vi "Periodic Tasks.vi"(8 "error in":errorcluster) -> ()   [LabVIEW 2018]
doc: "This VI runs in parallel to other tasks. It can contain as many user-defined periodic loops as you need. These can carry out PID or other sorts of timed response."
uses:
  PWF_Venom_LabVIEW/Public/TypeDefs/PwF_Venom_PIDParams.ctl
  DriveVenomDevRefs.ctl
  <vilib>/Rock Robotics/WPI/MotorControl/WPI_MotorControlDeviceRef.ctl
  <vilib>/Rock Robotics/WPI/MotorControl/WPI_MotorControlType.ctl
  <vilib>/Rock Robotics/SystemInterfaces/DIO/FPGA_DIOPWMChannel.ctl
  <vilib>/Rock Robotics/WPI/PWM/WPI_PWMDeadband.ctl
  <vilib>/Rock Robotics/SystemInterfaces/DIO/FPGA_DIOChannel.ctl
  DriveState.ctl
  PWF_Venom_LabVIEW/Public/TypeDefs/PwF_Venom_ControlMode.ctl
  88a8256b-dd6c-4d38-b021-9946be483166.vi
  72a4271e-8a2f-4e63-bef0-ab0047b3c302.vi
  4419bb08-cace-4eec-81e3-431b0f19f77f.vi
  43bb15c8-37b4-49b3-9761-3a694f89d06e.vi
  681b6e5e-4677-4682-a16d-7f94549bf0f7.vi
  f8245736-c666-4745-b76e-80ca56998d75.vi
  eff852b5-78a3-4797-aee6-6215f14f6dac.vi
  <vilib>/Array/Sort 2D Array - Pop Stack.vi
  <vilib>/Array/Sort 2D Array - Push Stack.vi
  <vilib>/Rock Robotics/WPI/Utilities/WPI_GetSetVariantRefNum.vi
  <vilib>/Rock Robotics/WPI/ThirdParty/Phoenix-LabVIEW/Pigeon IMU/CTRE_PigeonIMU_GetFusedHeading.vi
  <vilib>/Rock Robotics/Network Tables/NT Read Numeric Array.vi
  PWF_Venom_LabVIEW/PwF_Venom.lvlib
panel:
  in  "Set Angle":dbl(slide) scale=-180.0..180.0
  out "Degrees Off":dbl
  out "Center":dbl
  out "Height":dbl
  in  "Offset":dbl=182.0
  out "Waveform Chart":dbl(graph)=-0.0
  in  "PID Params":T1={"kP"=0.5, "kI"=0.0, "kD"=0.0, "kF"=0.184, "b"=0.0}
  in  "Track Width":dbl=2.3125
  in  "Tuning":dbl=10.0
  in  "Min Turn Radius":dbl=1.0
  in  "Max Wheel Velocity":dbl=4.0
  out "Avg Left Encoder (ft/s)":dbl
  out "Left Encoder (ft/s)":dbl
  in  "MinPower":dbl=0.063 format="%#_13g"
  out "dTime":u32=31
  out "Speed":dbl
  out "Position":dbl=-0.008333333333333333
  out "XY Graph":cluster{dbl[], dbl[]}(graph)
  out "RightEncoderInches":dbl=0.005423177083333334
  out "LeftEncoderInches":dbl=0.037962239583333335
  out "RightEncoderRaw":dbl=0.25
  out "LeftEncoderRaw":dbl=1.75
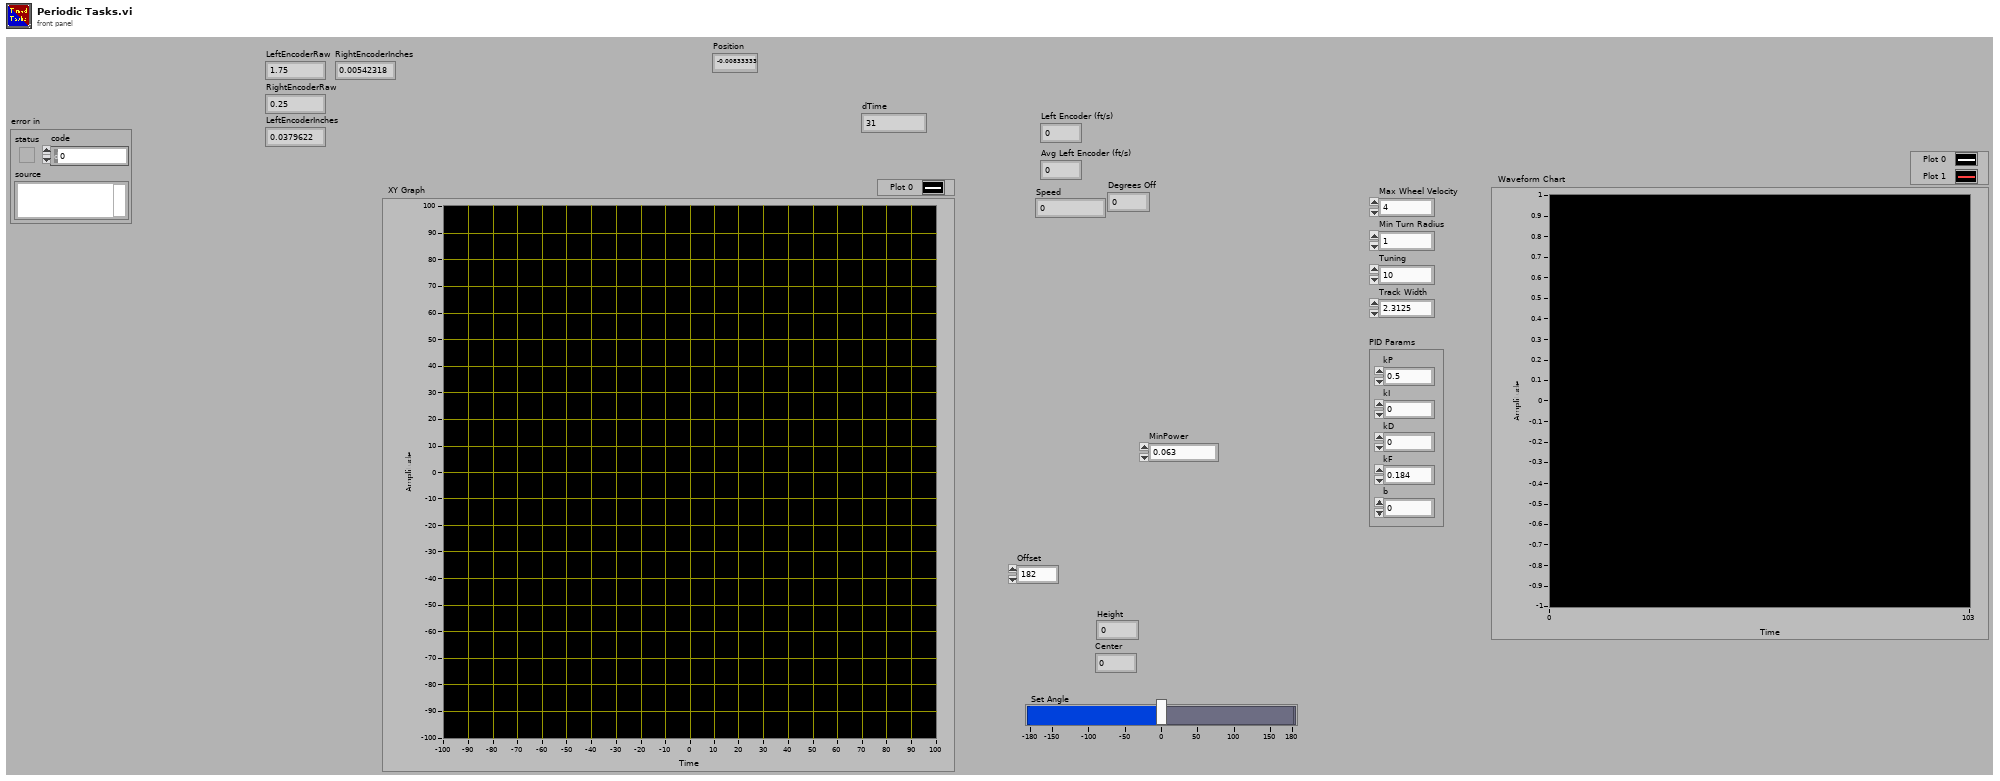
[diagram p1: front panel]
types:
  T1 = typedef "PwF_Venom.lvlib/PwF_Venom_PIDParams.ctl" = cluster{"kP":dbl, "kI":dbl, "kD":dbl, "kF":dbl, "b":dbl}
  T2 = cluster{"millisecond timer value":u32, "Distance":dbl}
  T3 = typedef "DriveVenomDevRefs.ctl" = cluster{"FrontLeft":T4, "FrontRight":T4}
  T4 = typedef "WPI_MotorControlDeviceRef.ctl" = cluster{"DeviceStatus":errorcluster, "Type":T5, "PWM":cluster{"PWM Channel":T6, "DeadBand":T7}, "CAN":cluster{"Device Number":u8, "SetOutput VI Ref":variant, "GetOutput VI Ref":variant, "Enable VI Ref":variant, "Disable VI Ref":variant, "Data":variant}, "Invert":bool, "DIO PWM":cluster{"PWM \"Enable\" Channel":T6, "DIOChannel":T8, "PWM Rate":dbl}}
  T5 = typedef "WPI_MotorControlType.ctl" = enum16{"PWM", "CAN", "DIO PWM"}
  T6 = typedef "FPGA_DIOPWMChannel.ctl" = enum8{"PWM 0", "PWM 1", "PWM 2", "PWM 3", "PWM 4", "PWM 5", "PWM 6", "PWM 7", "PWM 8", "PWM 9", "PWM MXP 0", "PWM MXP 1", "PWM MXP 2", "PWM MXP 3", "PWM MXP 4", "PWM MXP 5", "PWM MXP 6", "PWM MXP 7", "PWM MXP 8", "PWM MXP 9", "Invalid"}
  T7 = typedef "WPI_PWMDeadband.ctl" = cluster{"Name":string, "maxPositivePwm":i32, "minPositivePwm":i32, "centerPwm":i32, "maxNegativePwm":i32, "minNegativePwm":i32, "angularRange":u16}
  T8 = typedef "FPGA_DIOChannel.ctl" = enum8{"DIO 0", "DIO 1", "DIO 2", "DIO 3", "DIO 4", "DIO 5", "DIO 6", "DIO 7", "DIO 8", "DIO 9", "DIO MXP 0", "DIO MXP 1", "DIO MXP 2", "DIO MXP 3", "DIO MXP 4", "DIO MXP 5", "DIO MXP 6", "DIO MXP 7", "DIO MXP 8", "DIO MXP 9", "DIO MXP 10", "DIO MXP 11", "DIO MXP 12", "DIO MXP 13", "DIO MXP 14", "DIO MXP 15", "SPI Port CS1", "SPI Port CS2", "SPI Port CS3", "SPI Port MISO", "SPI Port MOSI", "Invalid"}
  T9 = typedef "WPI_I2CDevRef.ctl" = cluster{"DevStatus":errorcluster, "Device Address":u8, "Handle":i32, "I2C Bus":T10}
  T10 = typedef "i2c_bus.ctl" = enum16{"I2C On-Board", "I2C MXP", "Invalid"}
  T11 = typedef "CTRE_PigeonIMU_DeviceRef.ctl" = cluster{"DeviceStatus":errorcluster, "Device Number":u8, "Type":T12, "Device ID":u32, "Handle":u64, "UsageFrame":u32, "Library Path":path}
  T12 = typedef "CTRE_PigeonIMU_ConnectionType.ctl" = u32
  T13 = typedef "WPI_EncoderDevRef.ctl" = cluster{"DevStatus":errorcluster, "EncoderIndex":T14, "CounterIndex":T15, "DistancePerCount":dbl, "Decoding Type":T16}
  T14 = typedef "FPGA_EncoderIdx.ctl" = enum8{"Enc 0", "Enc 1", "Enc 2", "Enc 3", "Enc 4", "Enc 5", "Enc 6", "Enc 7", "Invalid"}
  T15 = typedef "FPGA_CounterCtrSystemIndex.ctl" = enum8{"Ctr 0", "Ctr 1", "Ctr 2", "Ctr 3", "Ctr 4", "Ctr 5", "Ctr 6", "Ctr 7", "Invalid"}
  T16 = typedef "WPI_EncoderType.ctl" = enum16{"1x", "2x", "4x"}
  T17 = typedef "WPI_JoystickDevRef.ctl" = cluster{"Device":T18}
  T18 = typedef "WPI_JoystickDeviceEnum.ctl" = enum16{"USB 0", "USB 1", "USB 2", "USB 3", "USB 4", "USB 5"}
  T19 = cluster{"millisecond timer value":u32, "Distance":dbl}[]
  T20 = enum16{"[0, 360]", "[-180, 180]", "[0, 2PI]", "[-PI, PI]"}
  T21 = cluster{"Heading":dbl, "Valid?":bool, "Fusing?":bool}
  T22 = typedef "DriveState.ctl" = enum16{"Manual", "Velocity", "Test Static Friction", "Do Nothing"}
  T23 = typedef "PwF_Venom.lvlib/PwF_Venom_ControlMode.ctl" = u8
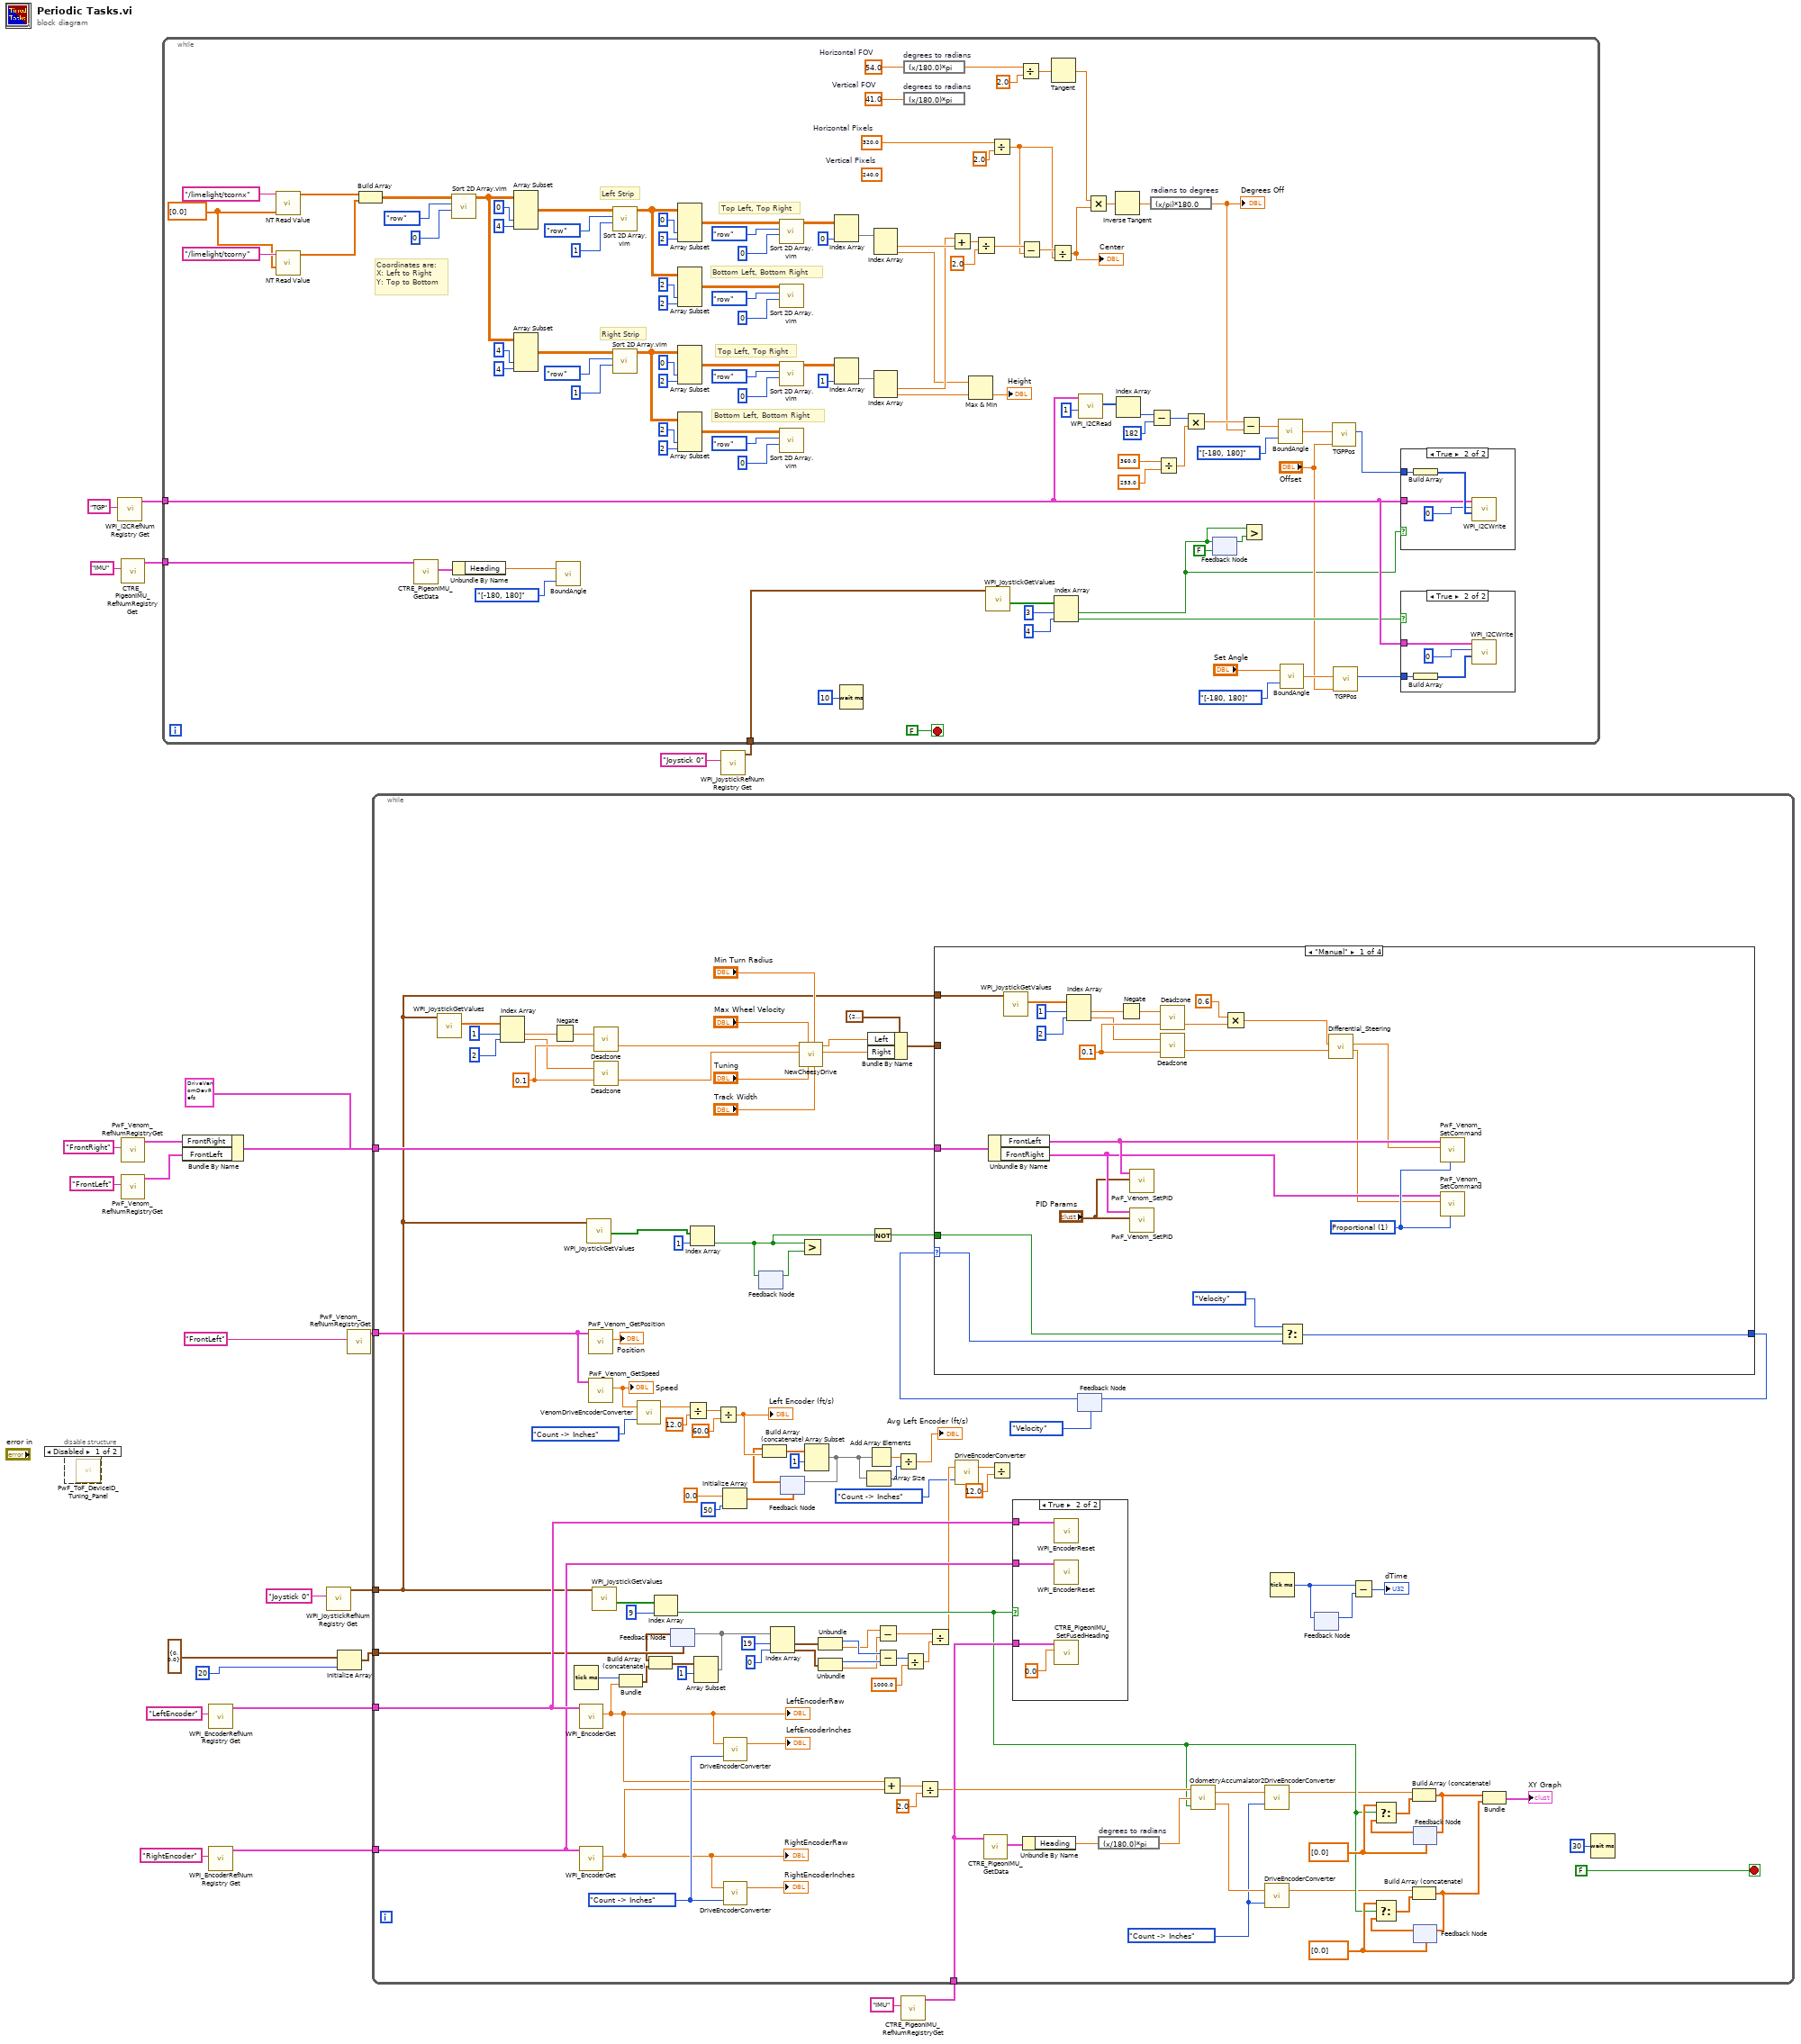
[diagram p0: block diagram]
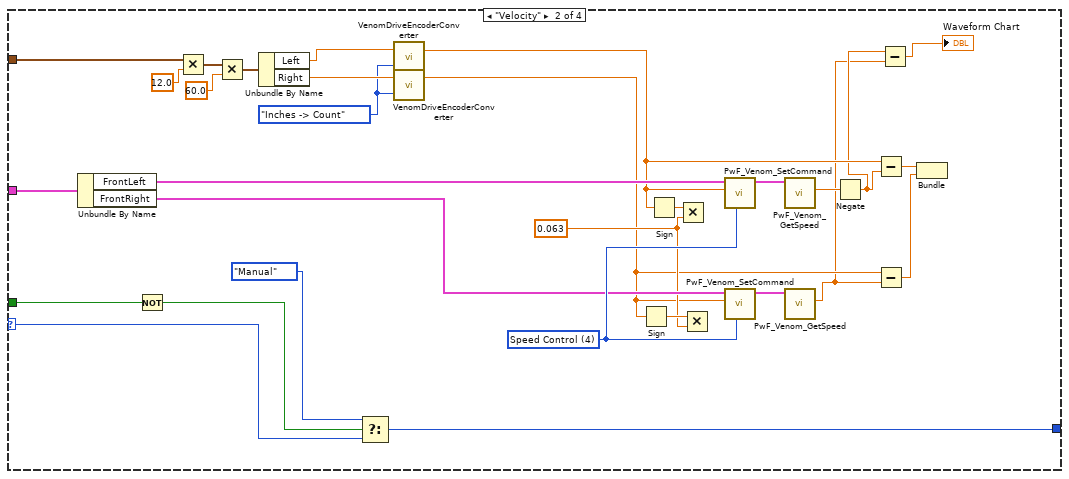
[diagram p6: hidden frame]
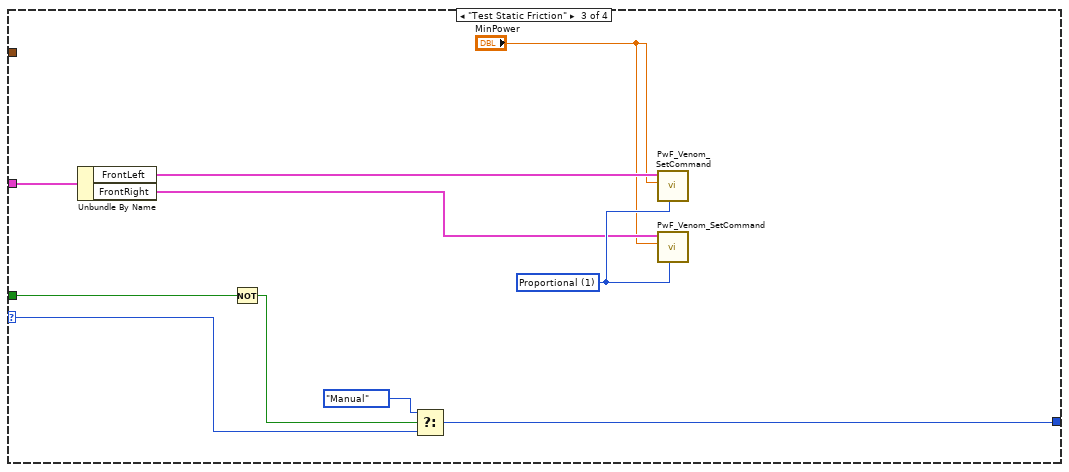
[diagram p7: hidden frame]
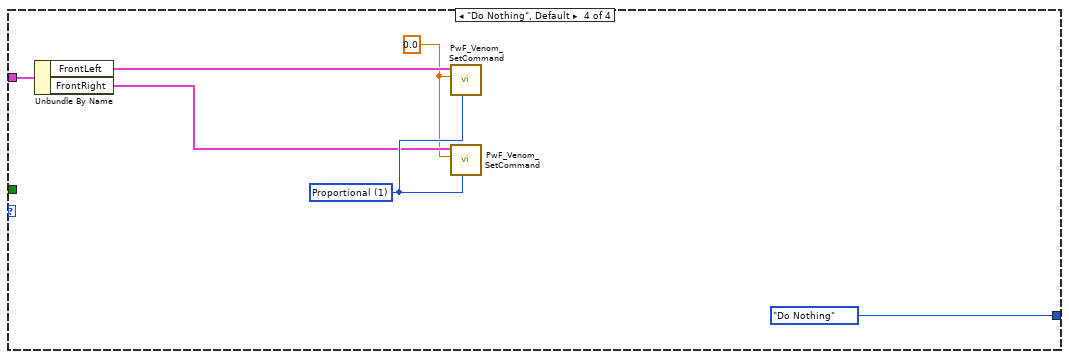
[diagram p8: hidden frame]
diagram:
  n1 = disable-structure shown="Disabled" {
    frame Disabled {
      n2 = call "PwF_ToF_DeviceID_Tuning_Panel.vi"() -> ()  [unwired: 12 in]
    }
    frame Enabled {
    }
  }
  n3 = call <vilib>:"WPI_I2CRefNum Registry Get.vi"("refnum name"="TGP") -> ("I2CDevRef"=w4:T9)  [unwired: 9 in, 1 out]
  n4 = call <vilib>:"CTRE_PigeonIMU_RefNumRegistryGet.vi"("refnum name"="IMU") -> ("PigeonIMUDevRef"=w3:T11)  [unwired: 9 in, 1 out]
  n5 = call "PwF_Venom_RefNumRegistryGet.vi"("refnum name"="FrontRight") -> ("PwFVenomDevRefOut"=w12:T4)  [unwired: 9 in, 1 out]
  n6 = call "PwF_Venom_RefNumRegistryGet.vi"("refnum name"="FrontLeft") -> ("PwFVenomDevRefOut"=w11:T4)  [unwired: 9 in, 1 out]
  n7 = Bundle By Name(cluster=T3 {"FrontLeft"={"DeviceStatus"={"status"=FALSE, "code"=0, "source"=""}, "Type"=enum."PWM", "PWM"={"PWM Channel"=enum."Invalid", "DeadBand"={"Name"="", "maxPositivePwm"=0, "minPositivePwm"=0, "centerPwm"=0, "maxNegativePwm"=0, "minNegativePwm"=0, "angularRange"=0}}, "CAN"={"Device Number"=0, "SetOutput VI Ref"=variant(refnum<vi> refnum), "GetOutput VI Ref"=variant(refnum<vi> refnum), "Enable VI Ref"=variant(refnum<vi> refnum), "Disable VI Ref"=variant(refnum<vi> refnum), "Data"=variant}, "Invert"=FALSE, "DIO PWM"={"PWM \"Enable\" Channel"=enum."Invalid", "DIOChannel"=enum."Invalid", "PWM Rate"=0.0}}, "FrontRight"={"DeviceStatus"={"status"=FALSE, "code"=0, "source"=""}, "Type"=enum."PWM", "PWM"={"PWM Channel"=enum."Invalid", "DeadBand"={"Name"="", "maxPositivePwm"=0, "minPositivePwm"=0, "centerPwm"=0, "maxNegativePwm"=0, "minNegativePwm"=0, "angularRange"=0}}, "CAN"={"Device Number"=0, "SetOutput VI Ref"=variant(refnum<vi> refnum), "GetOutput VI Ref"=variant(refnum<vi> refnum), "Enable VI Ref"=variant(refnum<vi> refnum), "Disable VI Ref"=variant(refnum<vi> refnum), "Data"=variant}, "Invert"=FALSE, "DIO PWM"={"PWM \"Enable\" Channel"=enum."Invalid", "DIOChannel"=enum."Invalid", "PWM Rate"=0.0}}} ("DriveVenomDevRefs"), "FrontRight"=w12, "FrontLeft"=w11) -> (w10:T3)
  n8 = call <vilib>:"WPI_EncoderRefNum Registry Get.vi"("refnum name"="LeftEncoder") -> ("EncoderDevRef"=w24:T13)  [unwired: 9 in, 1 out]
  n9 = call <vilib>:"WPI_EncoderRefNum Registry Get.vi"("refnum name"="RightEncoder") -> ("EncoderDevRef"=w23:T13)  [unwired: 9 in, 1 out]
  n10 = call <vilib>:"WPI_JoystickRefNum Registry Get.vi"("refnum name"="Joystick 0") -> ("JoystickDevRef"=w18:T17)  [unwired: 9 in, 1 out]
  n11 = Initialize Array(T2 {"millisecond timer value"=0, "Distance"=0.0}, 20 ("dimension size")) -> (w7:T19)
  n12 = call "PwF_Venom_RefNumRegistryGet.vi"("refnum name"="FrontLeft") -> ("PwFVenomDevRefOut"=w17:T4)  [unwired: 9 in, 1 out]
  n13 = call <vilib>:"WPI_JoystickRefNum Registry Get.vi"("refnum name"="Joystick 0") -> ("JoystickDevRef"=w1:T17)  [unwired: 9 in, 1 out]
  n14 = while {
    tunnel: w4 -> [w43]
    tunnel: w3 -> [w121]
    tunnel: w1 -> [w32]
    stop <- FALSE stop-if-true
    (unwired) 240.0  # Vertical Pixels
    w56 = 320.0  # Horizontal Pixels
    w65 = 41.0  # Vertical FOV
    w68 = 54.0  # Horizontal FOV
    w116 = dbl[] [0.0] ("Default Value")
    # "Coordinates are:\nX: Left to Right\nY: Top to Bottom"
    # "Top Left, Top Right"
    # "Bottom Left, Bottom Right"
    # "Top Left, Top Right"
    # "Bottom Left, Bottom Right"
    # "Right Strip"
    # "Left Strip"
    n15 = call-poly <vilib>:"NT Read Value.vi"("Default Value"=w116, "Name"="/limelight/tcornx") -> ("Numeric Array"=w118:dbl[])  [unwired: 8 in, 1 out]
    n16 = call-poly <vilib>:"NT Read Value.vi"("Default Value"=w116, "Name"="/limelight/tcorny") -> ("Numeric Array"=w117:dbl[])  [unwired: 8 in, 1 out]
    n17 = Build Array(w118, w117) -> (w113:dbl[][])
    n18 = call-poly <vilib>:"CTRE_PigeonIMU_GetData.vi"("PigeonIMUDevRef"=w121) -> ("Fused Heading"=w123:T21)  [unwired: 8 in, 2 out]
    n19 = call "Sort 2D Array.vim"("index"=0, "dimension to index (column)"=enum16{"column", "row"}."row", "2D array"=w113) -> ("sorted 2D array"=w108:dbl[][])  [unwired: 7 in, 1 out]
    n20 = Unbundle By Name(w123) -> ("Heading"=w124:dbl)
    n21 = Array Subset(array=w108, index (col)=0 ("index"), length (col)=4 ("index")) -> (w105:dbl[][])  [unwired: 2 in]
    n22 = Array Subset(array=w108, index (col)=4 ("index"), length (col)=4 ("index")) -> (w102:dbl[][])  [unwired: 2 in]
    n23 = call <userlib>:"BoundAngle.vi"("Type"=T20."[-180, 180]", "Angle"=w124) -> ()  [unwired: 1 out]
    n24 = call "Sort 2D Array.vim"("index"=1, "dimension to index (column)"=enum16{"column", "row"}."row", "2D array"=w105) -> ("sorted 2D array"=w97:dbl[][])  [unwired: 7 in, 1 out]
    n25 = call "Sort 2D Array.vim"("index"=1, "dimension to index (column)"=enum16{"column", "row"}."row", "2D array"=w102) -> ("sorted 2D array"=w92:dbl[][])  [unwired: 7 in, 1 out]
    n26 = Array Subset(array=w97, index (col)=0 ("index"), length (col)=2 ("index")) -> (w89:dbl[][])  [unwired: 2 in]
    n27 = Array Subset(array=w97, index (col)=2 ("index"), length (col)=2 ("index")) -> (w86:dbl[][])  [unwired: 2 in]
    n28 = Array Subset(array=w92, index (col)=0 ("index"), length (col)=2 ("index")) -> (w81:dbl[][])  [unwired: 2 in]
    n29 = Array Subset(array=w92, index (col)=2 ("index"), length (col)=2 ("index")) -> (w80:dbl[][])  [unwired: 2 in]
    n30 = call "Sort 2D Array.vim"("index"=0, "dimension to index (column)"=enum16{"column", "row"}."row", "2D array"=w89) -> ("sorted 2D array"=w77:dbl[][])  [unwired: 7 in, 1 out]
    n31 = call "Sort 2D Array.vim"("index"=0, "dimension to index (column)"=enum16{"column", "row"}."row", "2D array"=w86) -> ()  [unwired: 7 in, 2 out]
    n32 = call "Sort 2D Array.vim"("index"=0, "dimension to index (column)"=enum16{"column", "row"}."row", "2D array"=w81) -> ("sorted 2D array"=w76:dbl[][])  [unwired: 7 in, 1 out]
    n33 = call "Sort 2D Array.vim"("index"=0, "dimension to index (column)"=enum16{"column", "row"}."row", "2D array"=w80) -> ()  [unwired: 7 in, 2 out]
    n34 = Index Array(array=w77, index (col)=0 ("disabled index (col)")) -> (element=w75:dbl[])  [unwired: 1 in]
    n35 = Index Array(array=w76, index (col)=1 ("disabled index (col)")) -> (element=w74:dbl[])  [unwired: 1 in]
    n36 = Wait (ms)(milliseconds to wait=u32 10) -> ()  [unwired: 1 out]
    n37 = Index Array(array=w75) -> (element #1=w73:dbl, element #2=w71:dbl)  [unwired: 2 in]
    n38 = Index Array(array=w74) -> (element #1=w72:dbl, element #2=w70:dbl)  [unwired: 2 in]
    n39 = expression code="(x/180.0)*pi" "degrees to radians"(w68) -> (w66:dbl)
    n40 = expression code="(x/180.0)*pi" "degrees to radians"(w65) -> ()  [unwired: 1 out]
    n41 = Add(x=w72, y=w73) -> (x+y=w60:dbl)
    n42 = Max & Min(x=w71, y=w70) -> (min(x,y)=→"Height":dbl)  [unwired: 1 out]
    n43 = Divide(x=w60, y=2.0 ("x+y")) -> (x/y=w58:dbl)
    n44 = call <vilib>:"WPI_JoystickGetValues.vi"("JoystickDevRef"=w32) -> ("Buttons"=w37:bool[])  [unwired: 6 in, 4 out]
    n45 = Divide(x=w56, y=2.0) -> (x/y=w53:dbl)
    n46 = Divide(x=w66, y=2.0) -> (x/y=w64:dbl)
    n47 = Subtract(x=w58, y=w53) -> (x-y=w57:dbl)
    n48 = Divide(x=w57, y=w53) -> (x/y=w54:dbl)
    "Center" <- w54
    n49 = Tangent(1:w64) -> (0:w63:dbl)
    n50 = Index Array(array=w37, index #1=3 ("index"), index #2=4 ("index")) -> (element #1=w26:bool, element #2=w33:bool)
    n51 = call <vilib>:"WPI_I2CRead.vi"("I2CBytesToRead"=u8 1, "I2CDevRef"=w43) -> ("Data Out"=w52:u8[])  [unwired: 7 in, 2 out]
    n52 = Multiply(x=w63, y=w54) -> (x*y=w62:dbl)
    n53 = Inverse Tangent(1:w62) -> (0:w61:dbl)
    n54 = Index Array(array=w52) -> (element=w49:u8)  [unwired: 1 in]
    n55 = Subtract(x=w49, y=u8 182) -> (x-y=w29:u8)
    n56 = expression code="(x/pi)*180.0" "radians to degrees"(w61) -> (w30:dbl)
    "Degrees Off" <- w30
    n57 = Divide(x=360.0, y=253.0 ("x")) -> (x/y=w48:dbl)
    n58 = Multiply(x=w29, y=w48) -> (x*y=w31:dbl)
    n59 = feedback-in #1(w26) -> ()
    n60 = feedback #1(FALSE) -> (w35:bool)
    n61 = Subtract(x=w31, y=w30) -> (x-y=w46:dbl)
    n62 = Greater?(x=w26, y=w35) -> ()  [unwired: 1 out]
    n63 = call <userlib>:"BoundAngle.vi"("Type"=T20."[-180, 180]", "Angle"=w46) -> ("Bound Angle"=w45:dbl)
    n64 = call <userlib>:"BoundAngle.vi"("Type"=T20."[-180, 180]", "Angle"="Set Angle") -> ("Bound Angle"=w41:dbl)
    n65 = call "TGPPos.vi"("Offset"="Offset", "Angle (-179 - 180)"=w45) -> ("TGP Pos"=w44:u8)  [unwired: 9 in]
    n66 = call "TGPPos.vi"("Offset"="Offset", "Angle (-179 - 180)"=w41) -> ("TGP Pos"=w39:u8)  [unwired: 9 in]
    n67 = case shown="True" w26 {
      tunnel: w44 -> [_ w133]
      tunnel: w43 -> [_ w132]
      frame False {
      }
      frame True {
        n68 = Build Array(w133) -> (w135:u8[])
        n69 = call <vilib>:"WPI_I2CWrite.vi"("I2CDataToSend"=w135, "I2CRegister"=u8 0, "I2CDevRef"=w132) -> ()  [unwired: 7 in, 2 out]
      }
    }
    n70 = case shown="True" w33 {
      tunnel: w39 -> [_ w129]
      tunnel: w43 -> [_ w128]
      frame False {
      }
      frame True {
        n71 = Build Array(w129) -> (w131:u8[])
        n72 = call <vilib>:"WPI_I2CWrite.vi"("I2CDataToSend"=w131, "I2CRegister"=u8 0, "I2CDevRef"=w128) -> ()  [unwired: 7 in, 2 out]
      }
    }
  }
  n73 = call <vilib>:"CTRE_PigeonIMU_RefNumRegistryGet.vi"("refnum name"="IMU") -> ("PigeonIMUDevRef"=w20:T11)  [unwired: 9 in, 1 out]
  n74 = while {
    tunnel: w24 -> [w238]
    tunnel: w23 -> [w237]
    tunnel: w20 -> [w236]
    tunnel: w18 -> [w205]
    tunnel: w17 -> [w235]
    tunnel: w10 -> [w234]
    tunnel: w7 -> [w227]
    stop <- FALSE stop-if-true
    w176 = enum16{"Count -> Inches", "Inches -> Count"}."Count -> Inches" ("Mode")
    w190 = dbl[] [0.0]
    w191 = dbl[] [0.0]
    w204 = enum16{"Count -> Inches", "Inches -> Count"}."Count -> Inches" ("Mode")
    w214 = 0.1 ("Deadzone")
    n75 = call <vilib>:"WPI_JoystickGetValues.vi"("JoystickDevRef"=w205) -> ("Axes"=w215:dbl[])  [unwired: 6 in, 4 out]
    n76 = Index Array(array=w215, index #1=1 ("index"), index #2=2 ("index")) -> (element #1=w216:dbl, element #2=w210:dbl)
    n77 = Negate(x=w216) -> (-x=w211:dbl)
    n78 = Tick Count (ms)() -> (millisecond timer value=w170:u32)
    n79 = call <vilib>:"WPI_EncoderGet.vi"("EncoderDevRef"=w238) -> ("Distance"=w171:dbl)  [unwired: 5 in, 5 out]
    "LeftEncoderRaw" <- w171
    n80 = call <vilib>:"WPI_EncoderGet.vi"("EncoderDevRef"=w237) -> ("Distance"=w184:dbl)  [unwired: 5 in, 5 out]
    "RightEncoderRaw" <- w184
    n81 = call <vilib>:"WPI_JoystickGetValues.vi"("JoystickDevRef"=w205) -> ("Buttons"=w206:bool[])  [unwired: 6 in, 4 out]
    n82 = call "PwF_Venom_GetPosition.vi"("PwFVenomDevRefIn"=w235) -> ("Position"=→"Position":dbl)  [unwired: 8 in, 2 out]
    n83 = call "PwF_Venom_GetSpeed.vi"("PwFVenomDevRefIn"=w235) -> ("Speed"=w140:dbl)  [unwired: 8 in, 2 out]
    "Speed" <- w140
    n84 = call <vilib>:"WPI_JoystickGetValues.vi"("JoystickDevRef"=w205) -> ("Buttons"=w175:bool[])  [unwired: 6 in, 4 out]
    n85 = call <userlib>:"Deadzone.vi"("Deadzone"=w214, "Input Signal"=w211) -> ("Output Signal"=w209:dbl)  [unwired: 1 out]
    n86 = call <userlib>:"Deadzone.vi"("Deadzone"=w214, "Input Signal"=w210) -> ("Output Signal"=w208:dbl)  [unwired: 1 out]
    n87 = Bundle("millisecond timer value"=w170, "Distance"=w171) -> (w169:T2)  [unwired: 1 in]
    n88 = call "VenomDriveEncoderConverter.vi"("Mode"=enum16{"Count -> Inches", "Inches -> Count"}."Count -> Inches", "Input"=w140) -> ("Output"=w139:dbl)  [unwired: 1 in]
    n89 = Index Array(array=w175, index=9) -> (element=w185:bool)
    n90 = feedback #2(w227) -> (w172:T19)
    n91 = Build Array (concatenate)(w172, w169) -> (w174:T19)
    n92 = Divide(x=w139, y=12.0) -> (x/y=w137:dbl)
    n93 = Index Array(array=w206, index=1) -> (element=w228:bool)
    n94 = Array Subset(array=w174, index=1) -> (w168:T19)  [unwired: 1 in]
    n95 = feedback-in #2(w168) -> ()
    n96 = Divide(x=w137, y=60.0) -> (x/y=w226:dbl)
    "Left Encoder (ft/s)" <- w226
    n97 = Initialize Array(0.0 ("y"), 50 ("dimension size")) -> (w146:dbl[])
    n98 = call "DriveEncoderConverter.vi"("Mode"=w204, "Input"=w171) -> ("Output"=→"LeftEncoderInches":dbl)  [unwired: 1 in]
    n99 = call "DriveEncoderConverter.vi"("Mode"=w204, "Input"=w184) -> ("Output"=→"RightEncoderInches":dbl)  [unwired: 1 in]
    n100 = feedback-in #3(w228) -> ()
    n101 = feedback #3() -> (w229:bool)  [unwired: 1 in]
    n102 = Index Array(array=w168, index #1=19 ("index"), index #2=0 ("index")) -> (element #1=w165:T2, element #2=w164:T2)
    n103 = feedback #4(w146) -> (w149:dbl[])
    n104 = Build Array (concatenate)(w149, w226) -> (w151:dbl[])
    n105 = call "NewCheesyDrive.vi"("Track Width"="Track Width", "Min Turn Radius"="Min Turn Radius", "Tuning"="Tuning", "Max Wheel Velocity"="Max Wheel Velocity", "X"=w208, "Y"=w209) -> ("Right Speed"=w222:dbl, "Left Speed"=w221:dbl)  [unwired: 4 in]
    n106 = Greater?(x=w228, y=w229) -> ()  [unwired: 1 out]
    n107 = Array Subset(array=w151, index=1) -> (w145:dbl[])  [unwired: 1 in]
    n108 = feedback-in #4(w145) -> ()
    n109 = Unbundle(w165) -> ("millisecond timer value"=w163:u32, "Distance"=w161:dbl)
    n110 = Unbundle(w164) -> ("millisecond timer value"=w162:u32, "Distance"=w160:dbl)
    n111 = Array Size(array=w145) -> (size(s)=w143:i32)
    n112 = Bundle By Name(cluster=cluster{"Left":dbl, "Right":dbl} {"Left"=2.0, "Right"=2.0} ("input cluster"), "Left"=w221, "Right"=w222) -> (w223:cluster{"Left":dbl, "Right":dbl})
    n113 = Add Array Elements(numeric array=w145) -> (sum=w144:dbl)
    n114 = Not(x=w228) -> (.not. x?=w207:bool)
    n115 = Subtract(x=w161, y=w160) -> (x-y=w159:dbl)
    n116 = Subtract(x=w163, y=w162) -> (x-y=w154:u32)
    n117 = Add(x=w171, y=w184) -> (x+y=w201:dbl)
    n118 = Divide(x=w144, y=w143) -> (x/y=→"Avg Left Encoder (ft/s)":dbl)
    n119 = Divide(x=w154, y=1000.0) -> (x/y=w153:dbl)
    n120 = Divide(x=w201, y=2.0) -> (x/y=w199:dbl)
    n121 = Divide(x=w159, y=w153) -> (x/y=w158:dbl)
    n122 = call "DriveEncoderConverter.vi"("Mode"=enum16{"Count -> Inches", "Inches -> Count"}."Count -> Inches", "Input"=w158) -> ("Output"=w156:dbl)  [unwired: 1 in]
    n123 = call-poly <vilib>:"CTRE_PigeonIMU_GetData.vi"("PigeonIMUDevRef"=w236) -> ("Fused Heading"=w198:T21)  [unwired: 8 in, 2 out]
    n124 = Divide(x=w156, y=12.0) -> ()  [unwired: 1 out]
    n125 = case shown="True" w185 {
      tunnel: w238 -> [_ w244]
      tunnel: w237 -> [_ w243]
      tunnel: w236 -> [_ w242]
      frame False {
      }
      frame True {
        n126 = call <vilib>:"WPI_EncoderReset.vi"("EncoderDevRef"=w244) -> ()  [unwired: 9 in, 2 out]
        n127 = call <vilib>:"WPI_EncoderReset.vi"("EncoderDevRef"=w243) -> ()  [unwired: 9 in, 2 out]
        n128 = call <vilib>:"CTRE_PigeonIMU_SetFusedHeading.vi"("Value"=0.0, "PigeonIMUDevRef 2"=w242) -> ()  [unwired: 8 in, 2 out]
      }
    }
    n129 = Unbundle By Name(w198) -> ("Heading"=w195:dbl)
    n130 = feedback #5(DriveState."Velocity") -> (w232:T22)
    n131 = case shown="\"Manual\"" w232 {
      selector: w232 -> [w253 w292 w301 _]
      tunnel: w205 -> [w261 _ _ _]
      tunnel: w234 -> [w260 w296 w306 w312]
      tunnel: w223 -> [_ w283 _ _]
      tunnel: [w255 w293 w302 DriveState."Do Nothing"] -> w231
      tunnel: w207 -> [w254 w291 w300 _]
      frame "Manual" {
        w265 = 0.1 ("Deadzone")
        w264 = T23 1 items=["Disabled"=0, "Proportional"=1, "Current Control"=3, "Speed Control"=4, "Position Control"=5, "Motion Profile"=6, "Follow The Leader"=7, "Voltage Control"=8] ("PwF Venom Control Mode")
        n132 = Unbundle By Name(w260) -> ("FrontLeft"=w251:T4, "FrontRight"=w250:T4)
        n133 = call <vilib>:"WPI_JoystickGetValues.vi"("JoystickDevRef"=w261) -> ("Axes"=w266:dbl[])  [unwired: 6 in, 4 out]
        n134 = Index Array(array=w266, index #1=1 ("index"), index #2=2 ("index")) -> (element #1=w267:dbl, element #2=w257:dbl)
        n135 = Negate(x=w267) -> (-x=w259:dbl)
        n136 = call "PwF_Venom_SetPID.vi"("PID Params"="PID Params", "PwFVenomDevRefIn"=w251) -> ()  [unwired: 8 in, 2 out]
        n137 = call "PwF_Venom_SetPID.vi"("PID Params"="PID Params", "PwFVenomDevRefIn"=w250) -> ()  [unwired: 8 in, 2 out]
        n138 = call <userlib>:"Deadzone.vi"("Deadzone"=w265, "Input Signal"=w259) -> ("Output Signal"=w258:dbl)  [unwired: 1 out]
        n139 = call <userlib>:"Deadzone.vi"("Deadzone"=w265, "Input Signal"=w257) -> ("Output Signal"=w246:dbl)  [unwired: 1 out]
        n140 = Multiply(x=0.6, y=w258) -> (x*y=w245:dbl)
        n141 = Select(t=DriveState."Velocity", s=w254, f=w253) -> (s? t:f=w255:T22)
        n142 = call <userlib>:"Differential_Steering.vi"("Steer"=w246, "Base"=w245) -> ("Right"=w247:dbl, "Left"=w248:dbl)  [unwired: 4 in]
        n143 = call "PwF_Venom_SetCommand.vi"("PwF Venom Control Mode"=w264, "command"=w248, "PwFVenomDevRefIn"=w251) -> ()  [unwired: 7 in, 2 out]
        n144 = call "PwF_Venom_SetCommand.vi"("PwF Venom Control Mode"=w264, "command"=w247, "PwFVenomDevRefIn"=w250) -> ()  [unwired: 7 in, 2 out]
      }
      frame "Velocity" {
        w279 = enum16{"Count -> Inches", "Inches -> Count"}."Inches -> Count" ("Mode")
        w287 = 0.063
        w297 = T23 4 items=["Disabled"=0, "Proportional"=1, "Current Control"=3, "Speed Control"=4, "Position Control"=5, "Motion Profile"=6, "Follow The Leader"=7, "Voltage Control"=8] ("PwF Venom Control Mode")
        n145 = Unbundle By Name(w296) -> ("FrontLeft"=w295:T4, "FrontRight"=w294:T4)
        n146 = Not(x=w291) -> (.not. x?=w278:bool)
        n147 = Multiply(x=w283, y=12.0) -> (x*y=w285:cluster{"Left":dbl, "Right":dbl})
        n148 = Multiply(x=w285, y=60.0) -> (x*y=w282:cluster{"Left":dbl, "Right":dbl})
        n149 = Unbundle By Name(w282) -> ("Left"=w280:dbl, "Right"=w281:dbl)
        n150 = Select(t=DriveState."Manual", s=w278, f=w292) -> (s? t:f=w293:T22)
        n151 = call "VenomDriveEncoderConverter.vi"("Mode"=w279, "Input"=w280) -> ("Output"=w272:dbl)  [unwired: 1 in]
        n152 = call "VenomDriveEncoderConverter.vi"("Mode"=w279, "Input"=w281) -> ("Output"=w271:dbl)  [unwired: 1 in]
        n153 = Sign(1:w271) -> (0:w288:dbl)
        n154 = Sign(1:w272) -> (0:w289:dbl)
        n155 = Multiply(x=w289, y=w287) -> ()  [unwired: 1 out]
        n156 = Multiply(x=w288, y=w287) -> ()  [unwired: 1 out]
        n157 = call "PwF_Venom_SetCommand.vi"("PwF Venom Control Mode"=w297, "command"=w272, "PwFVenomDevRefIn"=w295) -> ("PwFVenomDevRefOut"=w273:T4)  [unwired: 7 in, 1 out]
        n158 = call "PwF_Venom_SetCommand.vi"("PwF Venom Control Mode"=w297, "command"=w271, "PwFVenomDevRefIn"=w294) -> ("PwFVenomDevRefOut"=w274:T4)  [unwired: 7 in, 1 out]
        n159 = call "PwF_Venom_GetSpeed.vi"("PwFVenomDevRefIn"=w273) -> ("Speed"=w277:dbl)  [unwired: 8 in, 2 out]
        n160 = call "PwF_Venom_GetSpeed.vi"("PwFVenomDevRefIn"=w274) -> ("Speed"=w269:dbl)  [unwired: 8 in, 2 out]
        n161 = Negate(x=w277) -> (-x=w270:dbl)
        n162 = Subtract(x=w272, y=w270) -> (x-y=w276:dbl)
        n163 = Subtract(x=w271, y=w269) -> (x-y=w275:dbl)
        n164 = Subtract(x=w270, y=w269) -> (x-y=→"Waveform Chart":dbl)
        n165 = Bundle(w276, w275) -> ()  [unwired: 1 in, 1 out]
      }
      frame "Test Static Friction" {
        w307 = T23 1 items=["Disabled"=0, "Proportional"=1, "Current Control"=3, "Speed Control"=4, "Position Control"=5, "Motion Profile"=6, "Follow The Leader"=7, "Voltage Control"=8] ("PwF Venom Control Mode")
        n166 = Unbundle By Name(w306) -> ("FrontLeft"=w305:T4, "FrontRight"=w304:T4)
        n167 = Not(x=w300) -> (.not. x?=w299:bool)
        n168 = Select(t=DriveState."Manual", s=w299, f=w301) -> (s? t:f=w302:T22)
        n169 = call "PwF_Venom_SetCommand.vi"("PwF Venom Control Mode"=w307, "command"="MinPower", "PwFVenomDevRefIn"=w305) -> ()  [unwired: 7 in, 2 out]
        n170 = call "PwF_Venom_SetCommand.vi"("PwF Venom Control Mode"=w307, "command"="MinPower", "PwFVenomDevRefIn"=w304) -> ()  [unwired: 7 in, 2 out]
      }
      frame "Do Nothing", Default {
        w309 = 0.0 ("command")
        w313 = T23 1 items=["Disabled"=0, "Proportional"=1, "Current Control"=3, "Speed Control"=4, "Position Control"=5, "Motion Profile"=6, "Follow The Leader"=7, "Voltage Control"=8] ("PwF Venom Control Mode")
        n171 = Unbundle By Name(w312) -> ("FrontLeft"=w311:T4, "FrontRight"=w310:T4)
        n172 = call "PwF_Venom_SetCommand.vi"("PwF Venom Control Mode"=w313, "command"=w309, "PwFVenomDevRefIn"=w311) -> ()  [unwired: 7 in, 2 out]
        n173 = call "PwF_Venom_SetCommand.vi"("PwF Venom Control Mode"=w313, "command"=w309, "PwFVenomDevRefIn"=w310) -> ()  [unwired: 7 in, 2 out]
      }
    }
    n174 = feedback-in #5(w231) -> ()
    n175 = expression code="(x/180.0)*pi" "degrees to radians"(w195) -> (w194:dbl)
    n176 = call "OdometryAccumalator2.vi"("Position"=w199, "Heading (rad)"=w194, "Reset?"=w185) -> ("X"=w178:dbl, "Y"=w180:dbl)  [unwired: 2 in]
    n177 = call "DriveEncoderConverter.vi"("Mode"=w176, "Input"=w178) -> ("Output"=w177:dbl)  [unwired: 1 in]
    n178 = call "DriveEncoderConverter.vi"("Mode"=w176, "Input"=w180) -> ("Output"=w179:dbl)  [unwired: 1 in]
    n179 = Tick Count (ms)() -> (millisecond timer value=w182:u32)
    n180 = feedback #6() -> (w183:u32)  [unwired: 1 in]
    n181 = feedback-in #6(w182) -> ()
    n182 = Subtract(x=w182, y=w183) -> (x-y=→"dTime":u32)
    n183 = feedback #7(w191) -> (w192:dbl[])
    n184 = Select(t=w191, s=w185, f=w192) -> (s? t:f=w193:dbl[])
    n185 = Build Array (concatenate)(w177, w193) -> (w197:dbl[])
    n186 = feedback-in #7(w197) -> ()
    n187 = feedback #8(w190) -> (w189:dbl[])
    n188 = Select(t=w190, s=w185, f=w189) -> (s? t:f=w188:dbl[])
    n189 = Build Array (concatenate)(w179, w188) -> (w186:dbl[])
    n190 = feedback-in #8(w186) -> ()
    n191 = Bundle(w197, w186) -> (→"XY Graph":cluster{dbl[], dbl[]})  [unwired: 1 in]
    n192 = Wait (ms)(milliseconds to wait=u32 30) -> ()  [unwired: 1 out]
  }
